vi "Read Write log to file.vi"(8 "error in (no error)":errorcluster, 11 "Errors in":refnum<class "CV-Errors.lvclass">) -> (0 "error out":errorcluster, 2 "Write log to file":bool, 3 "Errors out":refnum<class "CV-Errors.lvclass">)   [LabVIEW 2013, in "CameraVision.lvlib" / "CV-Errors.lvclass"]
uses:
  CV-Errors.lvclass
  CV-Errors.lvclass/CV-Errors.ctl
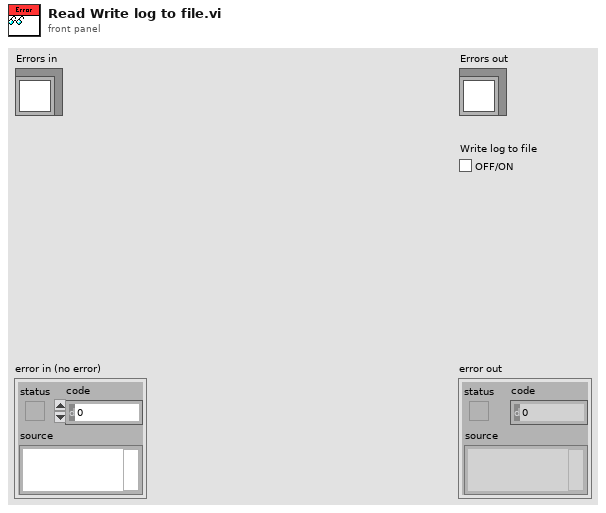
[diagram p1: front panel]
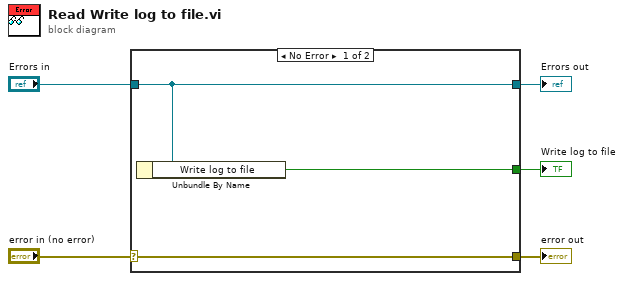
[diagram p0: block diagram]
diagram:
  n1 = case shown="No Error" "error in (no error)" {
    selector: "error in (no error)" -> [w8 w9]
    tunnel: [w8 w9] -> w4
    tunnel: [w7 w10] -> w2
    tunnel: "Errors in" -> [w7 w10]
    tunnel: [w6 _] -> w1
    frame No Error {
      n2 = Unbundle By Name(w7) -> ("Write log to file"=w6:bool)
    }
    frame Error {
    }
  }
  "error out" <- w4
  "Errors out" <- w2
  "Write log to file" <- w1
